vi "Transform Control Points.vi"(1 "ctrl pt":cluster{dbl, dbl}) -> (0 "ctrl pt out":cluster{dbl, dbl})   [LabVIEW 2019]
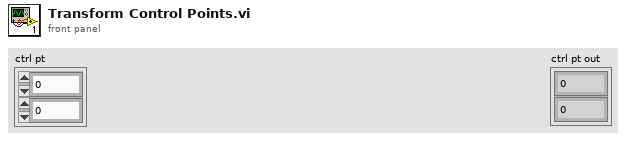
[diagram p1: front panel]
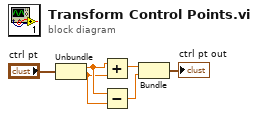
[diagram p0: block diagram]
diagram:
  n1 = Unbundle("ctrl pt") -> (w4:dbl, w3:dbl)
  n2 = Add(x=w4, y=w3) -> (x+y=w5:dbl)
  n3 = Subtract(x=w4, y=w3) -> (x-y=w2:dbl)
  n4 = Bundle(w5, w2) -> (→"ctrl pt out":cluster{dbl, dbl})  [unwired: 1 in]
